vi "Write Target Actor path.vi"(10 "Target Actor path":path, 11 "Message Scripter in":refnum<class "Message Scripter.lvclass">) -> (3 "Message Scripter out":refnum<class "Message Scripter.lvclass">)   [LabVIEW 2020, in "Message Maker.lvlib" / "Message Scripter.lvclass"]
uses:
  Message Scripter.lvclass
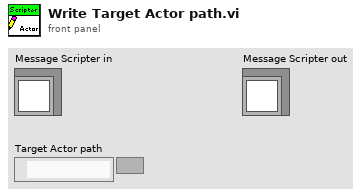
[diagram p1: front panel]
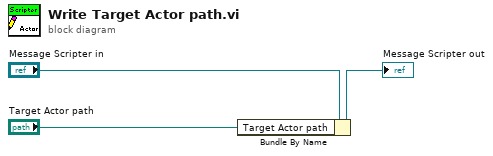
[diagram p0: block diagram]
diagram:
  n1 = Bundle By Name(cluster="Message Scripter in", "Target Actor path"="Target Actor path") -> (→"Message Scripter out":refnum<class "Message Scripter.lvclass">)
